vi "test Write File BIO.vi"(8 "error in (no error)":errorcluster, 11 "TestCase in":refnum<class "test BIO.lvclass">) -> (0 "error out":errorcluster, 3 "TestCase out":refnum<class "test BIO.lvclass">)   [LabVIEW 2013, in "test BIO.lvclass"]
uses:
  test BIO/test BIO.lvclass
  <vilib>/addons/_JKI Toolkits/VI Tester/TestCase.llb/TestCase.lvclass
  SSL_Lib/SSL-Lib/SSL-Lib.lvclass
  SSL_Lib/BIO/BIO.lvclass
  SSL_Lib/SSL-Lib/Library Paths.ctl
panel:
  out "return type":i32
  out "text":string
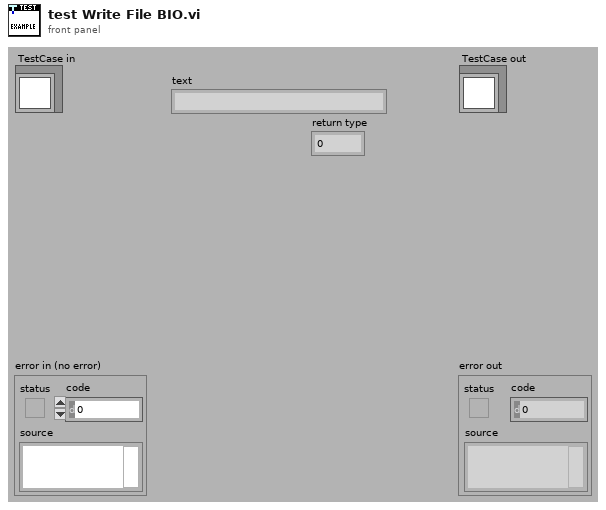
[diagram p1: front panel]
types:
  T1 = typedef "SSL_Lib.lvlib/SSL-Lib.lvclass/Library Paths.ctl" = cluster{"SSL Library Path":path, "Crypto Library Path":path}
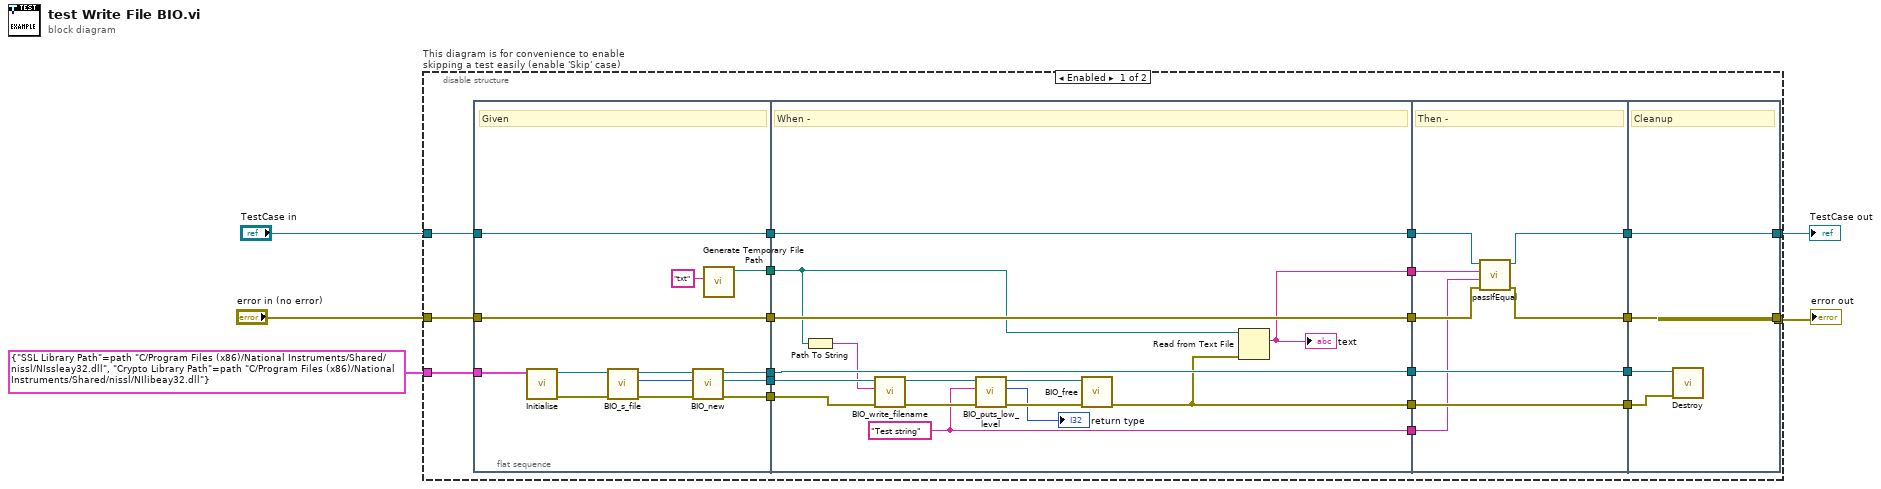
[diagram p0: block diagram]
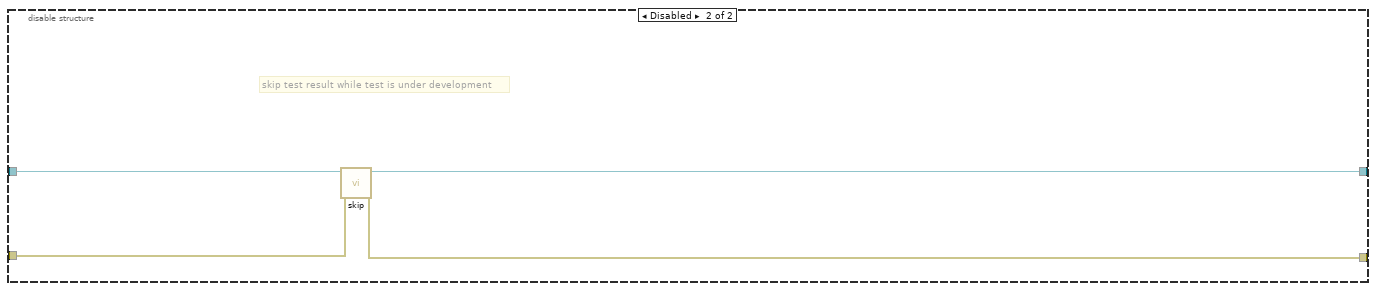
[diagram p2: hidden frame]
diagram:
  n1 = disable-structure "This diagram is for convenience to enable skipping a test easily (enable 'Skip' case)" shown="Enabled" {
    disable-tunnel: "TestCase in" -> [w19 w70]
    disable-tunnel: [w18 w68] -> w2
    disable-tunnel: [w17 w69] -> w4
    disable-tunnel: "error in (no error)" -> [w20 w67]
    disable-tunnel: T1 {"SSL Library Path"=path "C:/Program Files (x86)/National Instruments/Shared/nissl/NIssleay32.dll", "Crypto Library Path"=path "C:/Program Files (x86)/National Instruments/Shared/nissl/NIlibeay32.dll"} ("Library Paths") -> [w9 _]
    frame Enabled {
      n2 = flat-sequence {
        tunnel: w20 -> [w38]
        tunnel: w19 -> [w39]
        tunnel: [w39] -> w26
        tunnel: [w38] -> w25
        tunnel: [w32] -> w16
        tunnel: [w31] -> w15
        tunnel: [w30] -> w14
        tunnel: w9 -> [w29]
        tunnel: [w27] -> w8
        tunnel: [w54] -> w24
        tunnel: [w53] -> w23
        tunnel: w26 -> [w54]
        tunnel: w25 -> [w53]
        tunnel: w16 -> [w52]
        tunnel: w15 -> [w51]
        tunnel: w14 -> [w50]
        tunnel: [w50] -> w12
        tunnel: [w40] -> w10
        tunnel: w8 -> [w49]
        tunnel: [w47] -> w7
        tunnel: [w42] -> w6
        tunnel: [w61] -> w22
        tunnel: [w59] -> w21
        tunnel: w24 -> [w62]
        tunnel: w23 -> [w60]
        tunnel: [w58] -> w13
        tunnel: w12 -> [w58]
        tunnel: [w57] -> w11
        tunnel: w10 -> [w57]
        tunnel: w7 -> [w56]
        tunnel: w6 -> [w55]
        tunnel: [w65] -> w17
        tunnel: [w66] -> w18
        tunnel: w22 -> [w66]
        tunnel: w21 -> [w65]
        tunnel: w13 -> [w64]
        tunnel: w11 -> [w63]
        frame #0 {
          # "Given"
          n3 = call "Initialise.vi"("Library Paths"=w29) -> ("error out"=w34:errorcluster, "SSL-Lib out"=w35:refnum<class "SSL-Lib.lvclass">)  [unwired: 9 in]
          n4 = call "BIO_s_file.vi"("error in (no error)"=w34, "SSL-Lib in"=w35) -> ("error out"=w37:errorcluster, "*BIO_Method"=w33:u64, "SSL-Lib out"=w36:refnum<class "SSL-Lib.lvclass">)  [unwired: 7 in]
          n5 = call "BIO_new.vi"("error in (no error)"=w37, "*BIO_method"=w33, "SSL-Lib in"=w36) -> ("error out"=w31:errorcluster, "BIO out"=w32:refnum<class "BIO.lvclass">, "SSL-Lib out"=w30:refnum<class "SSL-Lib.lvclass">)  [unwired: 6 in]
          n6 = call <vilib>:"Generate Temporary File Path.vi"("Temporary File Extension (tmp)"="txt") -> ("Unique Temporary File Path"=w27:path)  [unwired: 9 in, 1 out]
        }
        frame #1 {
          w42 = "Test string" ("String to write")
          # "When -"
          n7 = Path To String(path=w49) -> (string=w48:string)
          n8 = call "BIO_write_filename.vi"("error in (no error)"=w51, "File path"=w48, "BIO in"=w52) -> ("error out"=w46:errorcluster, "BIO out"=w44:refnum<class "BIO.lvclass">)  [unwired: 7 in]
          n9 = call "BIO_puts_low_level.vi"("error in (no error)"=w46, "String to write"=w42, "BIO in"=w44) -> ("error out"=w45:errorcluster, "return type"=→"return type":i32, "BIO out"=w43:refnum<class "BIO.lvclass">)  [unwired: 6 in]
          n10 = call "BIO_free.vi"("error in (no error)"=w45, "BIO in"=w43) -> ("error out"=w40:errorcluster)  [unwired: 8 in, 1 out]
          n11 = Read from Text File(file (use dialog)=w49, error in=w40) -> (text=w47:string)  [unwired: 2 in, 3 out]
          "text" <- w47
        }
        frame #2 {
          # "Then -"
          n12 = call-dynamic "passIfEqual.vi"("error in (no error)"=w60, "y"=w55, "x"=w56, "TestCase in"=w62) -> ("error out"=w59:errorcluster, "TestCase out"=w61:refnum<class "test BIO.lvclass">)  [unwired: 6 in]
        }
        frame #3 {
          # "Cleanup"
          n13 = call "Destroy.vi"("error in (no error)"=w63, "SSL-Lib in"=w64) -> ()  [unwired: 9 in, 1 out]
        }
      }
    }
    frame Disabled {
      # "skip test result while test is under development"
      n14 = call <vilib>:"skip.vi"("error in (no error)"=w67, "TestCase in"=w70) -> ("error out"=w69:errorcluster, "TestCase out"=w68:refnum<class "test BIO.lvclass">)  [unwired: 8 in]
    }
  }
  "error out" <- w4
  "TestCase out" <- w2
